vi "Take_2_Pics.vi"(9 "Image Src Dark":T1, 10 "Image Src Light":T1, 11 "CameraDevRef":T2) -> (1 "Image Out Dark":T1, 2 "Image Out Light":T1)   [LabVIEW 2012]
uses:
  <vilib>/Rock Robotics/WPI/Camera/WPI_CameraDevRef.ctl
  <vilib>/vision/Image Controls.llb/IMAQ Image.ctl
  <vilib>/Rock Robotics/WPI/Relay/WPI_RelayValue.ctl
panel:
  in  "Milsec Wait":u32=80
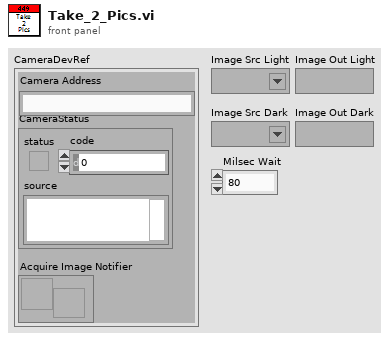
[diagram p1: front panel]
types:
  T1 = typedef "IMAQ Image.ctl" = refnum<image>
  T2 = typedef "WPI_CameraDevRef.ctl" = cluster{"Camera Address":string, "CameraStatus":errorcluster, "Acquire Image Notifier":refnum<notifier>}
  T3 = typedef "WPI_RelayValue.ctl" = enum16{"Off", "On", "Forward", "Reverse"}
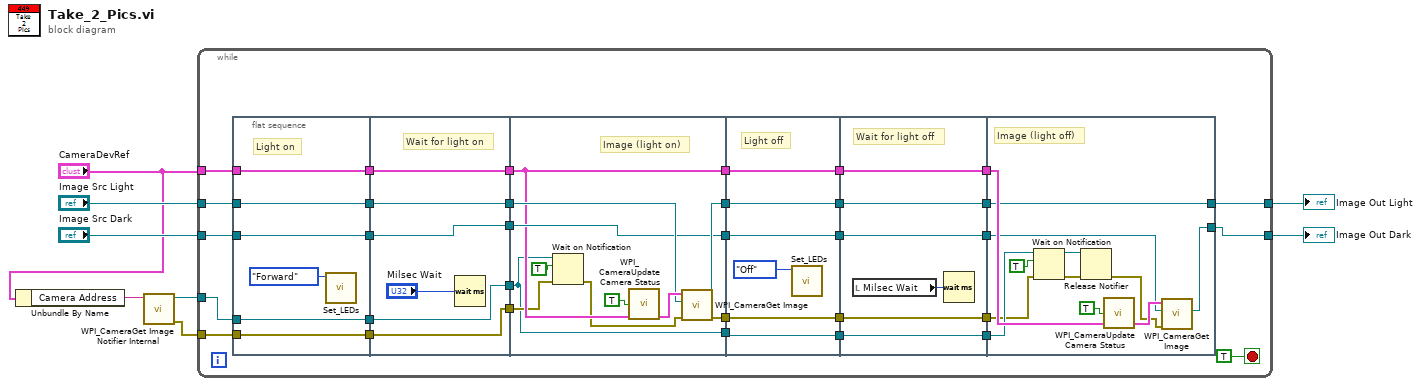
[diagram p0: block diagram]
diagram:
  n1 = Unbundle By Name("CameraDevRef") -> ("Camera Address"=w4:string)
  n2 = call <vilib>:"WPI_CameraGet Image Notifier Internal.vi"("Camera Address"=w4) -> ("error out"=w1:errorcluster, "Image Notifier"=w2:refnum<notifier>)  [unwired: 9 in]
  n3 = while {
    tunnel: "CameraDevRef" -> [w41]
    tunnel: "Image Src Light" -> [w40]
    tunnel: "Image Src Dark" -> [w27]
    tunnel: [w24] -> w5
    tunnel: [w23] -> w6
    tunnel: w2 -> [w17]
    tunnel: w1 -> [w13]
    stop <- TRUE stop-if-true
    n4 = flat-sequence {
      tunnel: w41 -> [w46]
      tunnel: w40 -> [w45]
      tunnel: [w46] -> w35
      tunnel: [w45] -> w33
      tunnel: [w44] -> w28
      tunnel: w27 -> [w44]
      tunnel: w17 -> [w43]
      tunnel: [w43] -> w16
      tunnel: [w42] -> w14
      tunnel: w13 -> [w42]
      tunnel: [w51] -> w36
      tunnel: w35 -> [w51]
      tunnel: [w53] -> w34
      tunnel: w33 -> [w53]
      tunnel: [w52] -> w29
      tunnel: w28 -> [w52]
      tunnel: [w49] -> w20
      tunnel: w16 -> [w49]
      tunnel: [w48] -> w15
      tunnel: w14 -> [w48]
      tunnel: [w59] -> w37
      tunnel: w36 -> [w59]
      tunnel: w34 -> [w62]
      tunnel: [w61] -> w32
      tunnel: [w60] -> w30
      tunnel: w29 -> [w60]
      tunnel: w20 -> [w54]
      tunnel: [w54] -> w19
      tunnel: w15 -> [w57]
      tunnel: [w55] -> w11
      tunnel: [w70] -> w38
      tunnel: w37 -> [w70]
      tunnel: w32 -> [w67]
      tunnel: [w69] -> w31
      tunnel: w30 -> [w69]
      tunnel: [w67] -> w21
      tunnel: w19 -> [w66]
      tunnel: [w66] -> w18
      tunnel: w11 -> [w65]
      tunnel: [w65] -> w9
      tunnel: w38 -> [w76]
      tunnel: w31 -> [w75]
      tunnel: [w76] -> w26
      tunnel: [w75] -> w25
      tunnel: [w74] -> w22
      tunnel: w21 -> [w74]
      tunnel: w18 -> [w73]
      tunnel: [w73] -> w12
      tunnel: [w72] -> w10
      tunnel: w9 -> [w72]
      tunnel: w26 -> [w86]
      tunnel: w25 -> [w85]
      tunnel: [w84] -> w24
      tunnel: [w83] -> w23
      tunnel: w22 -> [w83]
      tunnel: w12 -> [w78]
      tunnel: w10 -> [w77]
      frame #0 {
        # "Light on"
        n5 = call "Set_LEDs.vi"("RelayValue"=WPI_RelayValue."Forward") -> ()  [unwired: 10 in, 1 out]
      }
      frame #1 {
        # "Wait for light on"
        n6 = Wait (ms)(milliseconds to wait="Milsec Wait") -> ()  [unwired: 1 out]
      }
      frame #2 {
        # "Image (light on)"
        n7 = Wait on Notification(notifier=w54, ignore previous (F)=TRUE, error in (no error)=w57) -> (error out=w56:errorcluster)  [unwired: 1 in, 3 out]
        n8 = call <vilib>:"WPI_CameraUpdate Camera Status.vi"("CameraDevRef In"=w59, "Enable Vision"=TRUE) -> ("CameraDevRef Out"=w64:T2)  [unwired: 3 in]
        n9 = call <vilib>:"WPI_CameraGet Image.vi"("error in (no error)"=w56, "Image"=w62, "CameraDevRef"=w64) -> ("error out"=w55:errorcluster, "Image Out"=w61:T1)  [unwired: 6 in, 1 out]
      }
      frame #3 {
        # "Light off"
        n10 = call "Set_LEDs.vi"("RelayValue"=WPI_RelayValue."Off") -> ()  [unwired: 10 in, 1 out]
      }
      frame #4 {
        # "Wait for light off"
        n11 = local read "Milsec Wait"() -> (w71:u32)
        n12 = Wait (ms)(milliseconds to wait=w71) -> ()  [unwired: 1 out]
      }
      frame #5 {
        # "Image (light off)"
        n13 = Wait on Notification(notifier=w78, ignore previous (F)=TRUE, error in (no error)=w77) -> (notifier out=w81:refnum<notifier>, error out=w82:errorcluster)  [unwired: 1 in, 2 out]
        n14 = Release Notifier(notifier=w81, error in (no error)=w82) -> (error out=w79:errorcluster)  [unwired: 1 in, 2 out]
        n15 = call <vilib>:"WPI_CameraUpdate Camera Status.vi"("CameraDevRef In"=w86, "Enable Vision"=TRUE) -> ("CameraDevRef Out"=w87:T2)  [unwired: 3 in]
        n16 = call <vilib>:"WPI_CameraGet Image.vi"("error in (no error)"=w79, "Image"=w85, "CameraDevRef"=w87) -> ("Image Out"=w84:T1)  [unwired: 6 in, 2 out]
      }
    }
  }
  "Image Out Light" <- w6
  "Image Out Dark" <- w5
